vi "Acquire high frequencies.vi"() -> ()   [LabVIEW 2010]
panel:
  out "ErrMsg":string="No error has occurred"
  out "ErrCode":i32
  out "Waveform Graph":u16[](graph)=[1632, 1632, 1638, 1636, 1640, 1642, 1644, 1646, 1650, 1652, 1656, 1658, 1658, 1662, 1664, 1666, 1670, 1672, 1674, 1676, 1678, 1680, 1686, 1686, 1680, 1690, 1694, 1696, 1700, 1700, 1704, 1708, 1708, 1712, 1714, 1716, 1720, 1720, 1724, 1726, 1730, 1732, 1738, 1736, 1740, 1740, 1744, 1748, 1750, 1754, 1754, 1756, 1760, 1762, 1768, 1766, 1770, 1772, 1774, 1778, 1780, 1782, 1786, 1788, 1790, 1792, 1790, 1798, 1800, 1802, 1810, 1810, 1810, 1814, 1818, 1820, 1822, 1822, 1830, 1830, 1832, 1834, 1838, 1840, 1844, 1844, 1848, 1850, 1846, 1854, 1858, 1860, 1864, 1868, 1868, 1872, 1874, 1876, 1878, 1882, 1884, 1888, 1890, 1892, 1896, 1898, 1902, 1902, 1906, 1910, 1912, 1912, 1914, 1920, 1922, 1924, 1928, 1928, 1934, 1934, 1936, 1942, 1942, 1944, 1948, 1950, 1954, 1956, 1958, 1962, 1964, 1966, 1968, 1972, 1976, 1976, 1982, 1982, 1982, 1988, 1990, 1992, 1996, 1998, 2006, 2004, 2010, 2010, 2014, 2014, 2018, 2020, 2026, 2026, 2028, 2030, 2036, 2036, 2040, 2042, 2044, 2046, 2050, 2052, 2054, 2056, 2060, 2062, 2066, 2068, 2070, 2074, 2080, 2078, 2082, 2084, 2086, 2090, 2094, 2094, 2096, 2100, 2102, 2104, 2108, 2110, 2112, 2116, 2118, 2120, 2124, 2126, 2128, 2132, 2134, 2136, 2142, 2142, 2146, 2148, 2150, 2152, 2158, 2158, 2162, 2164, 2168, 2168, 2172, 2174, 2178, 2180, 2176, 2184, 2188, 2188, 2192, 2196, 2198, 2200, 2202, 2204, 2210, 2210, 2212, 2216, 2222, 2220, 2218, 2226, 2228, 2232, 2234, 2238, 2240, 2242, 2248, 2246, 2250, 2252, 2254, 2258, 2260, 2262, 2266, 2268, 2270, 2272, 2276, 2278, 2280, 2282, 2286, 2290, 2292, 2294, 2292, 2298, 2302, 2302, 2304, 2306, 2310, 2312, 2318, 2316, 2322, 2322, 2326, 2326, 2330, 2334, 2336, 2338, 2340, 2342, 2346, 2348, 2350, 2354, 2356, 2358, 2360, 2362, 2366, 2366, 2370, 2372, 2378, 2376, 2382, 2382, 2384, 2388, 2390, 2392, 2394, 2398, 2400, 2402, 2402, 2406, 2410, 2412, 2414, 2416, 2420, 2422, 2424, 2426, 2430, 2430, 2436, 2434, 2438, 2440, 2442, 2444, 2446, 2450, 2450, 2454, 2458, 2458, 2462, 2462, 2466, 2468, 2470, 2472, 2474, 2478, 2480, 2480, 2484, 2486, 2490, 2492, 2490, 2494, 2498, 2500, 2502, 2504, 2506, 2510, 2516, 2512, 2516, 2518, 2520, 2522, 2524, 2526, 2530, 2530, 2534, 2534, 2538, 2540, 2542, 2544, 2546, 2548, 2550, 2552, 2558, 2558, 2560, 2558, 2562, 2564, 2568, 2568, 2570, 2572, 2576, 2576, 2580, 2582, 2588, 2584, 2588, 2590, 2592, 2594, 2594, 2598, 2600, 2602, 2604, 2606, 2608, 2610, 2612, 2614, 2614, 2616, 2620, 2622, 2622, 2624, 2630, 2628, 2628, 2630, 2636, 2636, 2638, 2638, 2638, 2644, 2644, 2646, 2650, 2650, 2654, 2654, 2656, 2656, 2660, 2662, 2662, 2664, 2668, 2668, 2672, 2670, 2674, 2676, 2676, 2678, 2682, 2682, 2684, 2686, 2686, 2688, 2690, 2690, 2696, 2694, 2696, 2698, 2700, 2700, 2702, 2704, 2704, 2708, 2710, 2710, 2710, 2714, 2716, 2718, 2718, 2718, 2722, 2720, 2724, 2726, 2726, 2730, 2730, 2732, 2734, 2734, 2736, 2738, 2738, 2740, 2742, 2742, 2744, 2746, 2746, 2748, 2750, 2750, 2750, 2752, 2756, 2754, 2758, 2758, 2764, 2760, 2760, 2762, 2766, 2766, 2766, 2766, 2770, 2770, 2770, 2772, 2776, 2774, 2778, 2776, 2778, 2780, 2780, 2782, 2784, 2782, 2786, 2786, 2788, 2788, 2790, 2788, 2790, 2794, 2794, 2794, 2796, 2796, 2796, 2798, 2798, 2798, 2802, 2802, 2802, 2804, 2798, 2804, 2808, 2806, 2808, 2808, 2810, 2810, 2812, 2812, 2808, 2814, 2814, 2814, 2816, 2816, 2820, 2818, 2818, 2818, 2822, 2822, 2822, 2822, 2824, 2824, 2826, 2826, 2828, 2826, 2828, 2828, 2830, 2830, 2830, 2830, 2832, 2832, 2834, 2834, 2834, 2836, 2836, 2834, 2838, 2836, 2838, 2838, 2838, 2838, 2840, 2840, 2842, 2842, 2842, 2844, 2846, 2844, 2844, 2846, 2844, 2846, 2846, 2846, 2848, 2848, 2848, 2848, 2848, 2848, 2850, 2850, 2850, 2852, 2848, 2850, 2850, 2848, 2848, 2846, 2846, 2844, 2846, 2842, 2844, 2842, 2842, 2840, 2840, 2838, 2838, 2836, 2834, 2836, 2836, 2832, 2832, 2830, 2830, 2830, 2828, 2826, 2828, 2826, 2824, 2824, 2822, 2822, 2820, 2820, 2818, 2814, 2820, 2814, 2814, 2812, 2812, 2810, 2810, 2806, 2806, 2804, 2804, 2802, 2800, 2798, 2798, 2794, 2794, 2794, 2790, 2790, 2790, 2786, 2786, 2782, 2782, 2780, 2780, 2778, 2774, 2774, 2776, 2770, 2770, 2766, 2766, 2764, 2762, 2758, 2758, 2756, 2756, 2752, 2750, 2750, 2748, 2744, 2742, 2742, 2744, 2736, 2736, 2732, 2732, 2730, 2726, 2726, 2724, 2718, 2718, 2716, 2714, 2710, 2710, 2708, 2704, 2702, 2700, 2698, 2696, 2692, 2692, 2688, 2688, 2684, 2680, 2678, 2678, 2674, 2668, 2670, 2666, 2662, 2662, 2658, 2654, 2654, 2650, 2650, 2644, 2642, 2640, 2636, 2632, 2632, 2630, 2626, 2624, 2622, 2618, 2614, 2608, 2610, 2608, 2606, 2602, 2598, 2596, 2592, 2592, 2586, 2586, 2580, 2578, 2576, 2572, 2568, 2568, 2564, 2560, 2556, 2556, 2552, 2548, 2544, 2542, 2540, 2538, 2532, 2534, 2526, 2524, 2518, 2516, 2514, 2510, 2506, 2504, 2500, 2496, 2494, 2490, 2488, 2486, 2482, 2478, 2476, 2474, 2466, 2466, 2460, 2458, 2454, 2452, 2448, 2444, 2440, 2438, 2434, 2430, 2428, 2422, 2420, 2418, 2414, 2410, 2406, 2404, 2400, 2398, 2394, 2386, 2386, 2382, 2380, 2376, 2372, 2368, 2366, 2364, 2358, 2354, 2350, 2350, 2342, 2340, 2334, 2334, 2330, 2326, 2322, 2322, 2314, 2312, 2308, 2304, 2302, 2296, 2294, 2292, 2284, 2284, 2280, 2276, 2272, 2268, 2262, 2262, 2256, 2252, 2250, 2246, 2244, 2238, 2236, 2224, 2226, 2224, 2220, 2216, 2212, 2208, 2204, 2202, 2198, 2192, 2190, 2188, 2182, 2182, 2174, 2166, 2170, 2166, 2158, 2158, 2152, 2150, 2144, 2142, 2138, 2134, 2128, 2126, 2122, 2116, 2114, 2110, 2108, 2104, 2100, 2096, 2092, 2090, 2084, 2080, 2076, 2074, 2070, 2066, 2062, 2060, 2052, 2052, 2048, 2042, 2038, 2038, 2030, 2028, 2024, 2020, 2016, 2006, 2008, 2000, 2002, 1998, 1992, 1986, 1986, 1986, 1978, 1974, 1972, 1968, 1962, 1962, 1956, 1952, 1950, 1942, 1940, 1938, 1934, 1930, 1924, 1922, 1918, 1918, 1910, 1908, 1904, 1898, 1896, 1892, 1888, 1886, 1880, 1878, 1874, 1870, 1866, 1860, 1858, 1856, 1852, 1846, 1844, 1840, 1838, 1832, 1830, 1826, 1822, 1818, 1814, 1812, 1806, 1804, 1800, 1796, 1792, 1790, 1786, 1782, 1780, 1776, 1772, 1768, 1764, 1760, 1756, 1754, 1748, 1746, 1742, 1740, 1734, 1732, 1728, 1720, 1722, 1718, 1712, 1710, 1706, 1702, 1698, 1696, 1692]
  in  "Range":i32(ring)=1 items=["Not Programmable"=0, "+- 20 V"=27, "+- 10 V"=1, "+- 5 V"=2, "+- 4 V"=28, "+- 2.5 V"=3, "+- 2 V"=29, "+- 1.67 V"=4, "+- 1.25 V"=5, "+- 1 V"=6, "+- .625 V"=7, "+- .5 V"=8, "+- .25 V"=30, "+- .2 V"=31, "+- .1 V"=9, "+- .05 V"=10, "+- .01 V"=11, "+- .005 V"=12, "0 - 10 V"=13, "0 - 5 V"=14, "0 - 4 V"=36, "0 - 2.5 V"=15, "0 - 2 V"=16, "0 - 1.67 V"=17, "0 - 1.25 V"=18, "0 - 1 V"=19, "0 - .5 V"=32, "0 - .25 V"=33, "0 - .2 V"=34, "0 - .1 V"=20, "0 - .02 V"=35, "0 - .01 V"=21, "4 - 20 mA"=22, "2 - 10 mA"=23, "1 - 5 mA"=24, ".5 - 2.5 mA"=25, "0 - 20 mA"=26]
  in  "Rate":i32=1000
  in  "Count":i32=1000
  in  "HighChan":i32=1
  in  "LowChan":i32=1
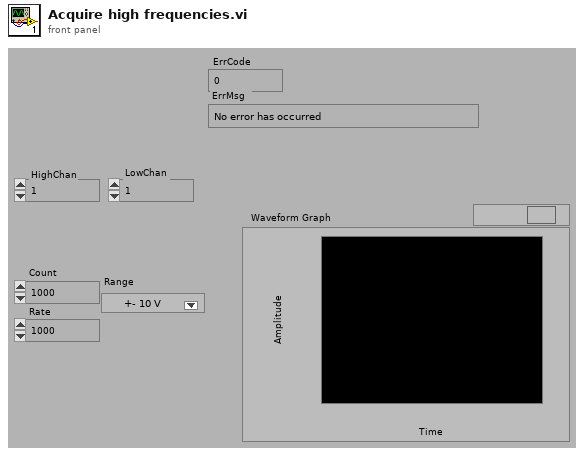
[diagram p1: front panel]
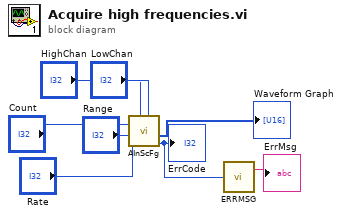
[diagram p0: block diagram]
diagram:
  n1 = call <menus>:"AInScFg.VI"("LowChan"="LowChan", "HighChan"="HighChan", "Range"="Range", "Rate"="Rate", "Count"="Count") -> ("ErrCode"=w2:i32, "ADData"=→"Waveform Graph":u16[])  [unwired: 3 in, 1 out]
  "ErrCode" <- w2
  n2 = call <menus>:"ERRMSG.VI"("ErrCode"=w2) -> ("ErrMsg"=→"ErrMsg":string)  [unwired: 1 out]
